vi "myRIO_BRig_RT_dataCurrent_laser2_tCue1_end.vi"() -> (2 "output_laser2_tCue1_end":i32)   [LabVIEW 2014]
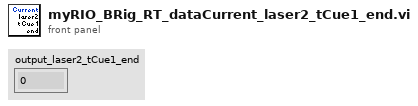
[diagram p1: front panel]
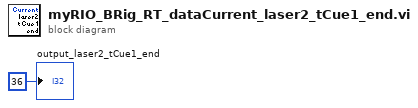
[diagram p0: block diagram]
diagram:
  "output_laser2_tCue1_end" <- 36 ("output_iBlock")
